vi "Chroma 1905x Series Get Data.vi"(0 "inst handle in":refnum<visa-resource-name>, 3 "error in":T1) -> (6 "inst handle out":refnum<visa-resource-name>, 7 "Status":string, 9 "error out":T1)   [LabVIEW 2025]
doc: "Chroma\n5 Clock Tower Place Suite 210\nMaynard, MA 01754\nTel: 1 800 253-1230\nTel: 1 877 4 A HIPOT\nFax: 1 978-461-4295\nWebsite: www.chroma.com"
uses:
  <instrlib>/Chroma 19052/Chroma 19052.lvlib
panel:
  out "read buffer":string
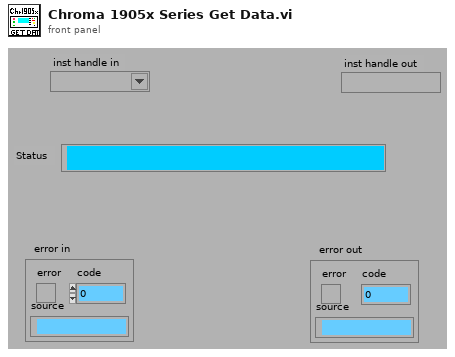
[diagram p1: front panel]
types:
  T1 = cluster{"error":bool, "code":i8, "source":string}
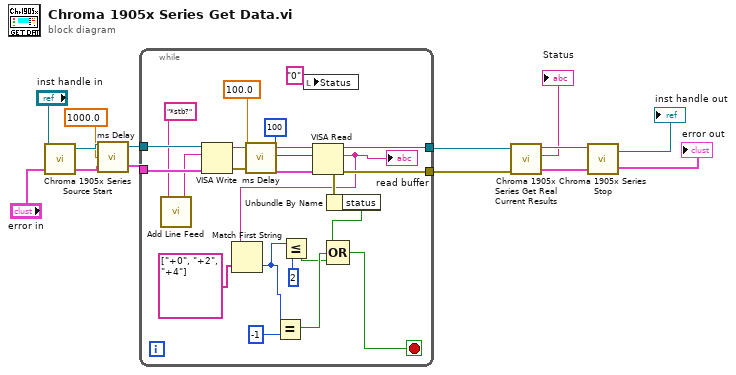
[diagram p0: block diagram]
diagram:
  n1 = call "Chroma 1905x Series Source Start.vi"("inst handle in"="inst handle in", "error in"="error in") -> ("inst handle out"=w5:refnum<visa-resource-name>, "error out"=w4:T1)  [unwired: 6 in]
  n2 = call <instrlib>:"ms Delay.vi"("error in"=w4, "Time Delay S"=1000.0, "inst handle in"=w5) -> ("error out"=w3:T1, "inst handle Out"=w2:refnum<visa-resource-name>)
  n3 = while {
    tunnel: [w32] -> w13
    tunnel: [w33] -> w14
    tunnel: w2 -> [w35]
    tunnel: w3 -> [w34]
    stop <- w31 stop-if-true
    n4 = call <instrlib>:"Add Line Feed.vi"("Cmdstring"="*stb?") -> ("Concatenated String"=w24:string)
    n5 = VISA Write(VISA resource name=w35, write buffer=w24, error in (no error)=w34) -> (VISA resource name out=w28:refnum<visa-resource-name>, error out=w29:errorcluster)  [unwired: 1 out]
    n6 = call <instrlib>:"ms Delay.vi"("error in"=w29, "Time Delay S"=100.0, "inst handle in"=w28) -> ("error out"=w26:T1, "inst handle Out"=w27:refnum<visa-resource-name>)
    n7 = local write "Status"("0" ("Status")) -> ()
    n8 = VISA Read(VISA resource name=w27, byte count=100, error in (no error)=w26) -> (VISA resource name out=w32:refnum<visa-resource-name>, read buffer=w22:string, error out=w33:errorcluster)  [unwired: 1 out]
    "read buffer" <- w22
    n9 = Match First String(2:string[] ["+0", "+2", "+4"] ("string array"), 3:w22) -> (0:w17:i32)  [unwired: 1 out]
    n10 = Equal?(x=w17, y=-1) -> (x = y?=w18:bool)
    n11 = Less Or Equal?(x=w17, y=2) -> (x <= y?=w15:bool)
    n12 = Unbundle By Name(w33) -> ("status"=w30:bool)
    n13 = Compound Arithmetic op=OR(w30, w18, w15) -> (w31:bool)
  }
  n14 = call "Chroma 1905x Series Get Real Current Results.vi"("inst handle Out"=w13, "error in"=w14) -> ("inst handle in"=w9:refnum<visa-resource-name>, "Result"=→"Status":string, "error out"=w12:T1)  [unwired: 1 in]
  n15 = call "Chroma 1905x Series Stop.vi"("error in"=w12, "inst handle in"=w9) -> ("error out"=→"error out":T1, "inst handle out"=→"inst handle out":refnum<visa-resource-name>)  [unwired: 1 in]
